vi "Image Version.vi"(6 "Flags":u32=65535 format="%.0x", 8 "error in":errorcluster) -> (0 "error out":errorcluster, 3 "Return":i32)   [LabVIEW 2014]
uses:
  DLL/SDL2.dll
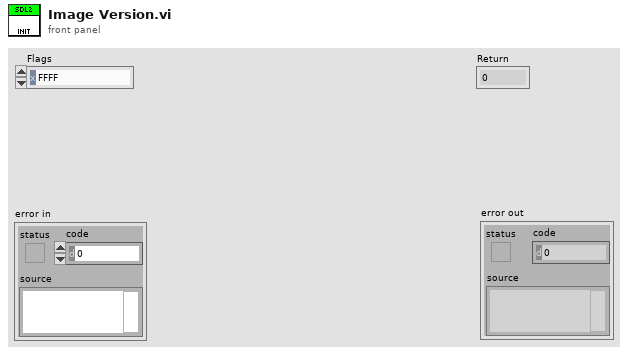
[diagram p1: front panel]
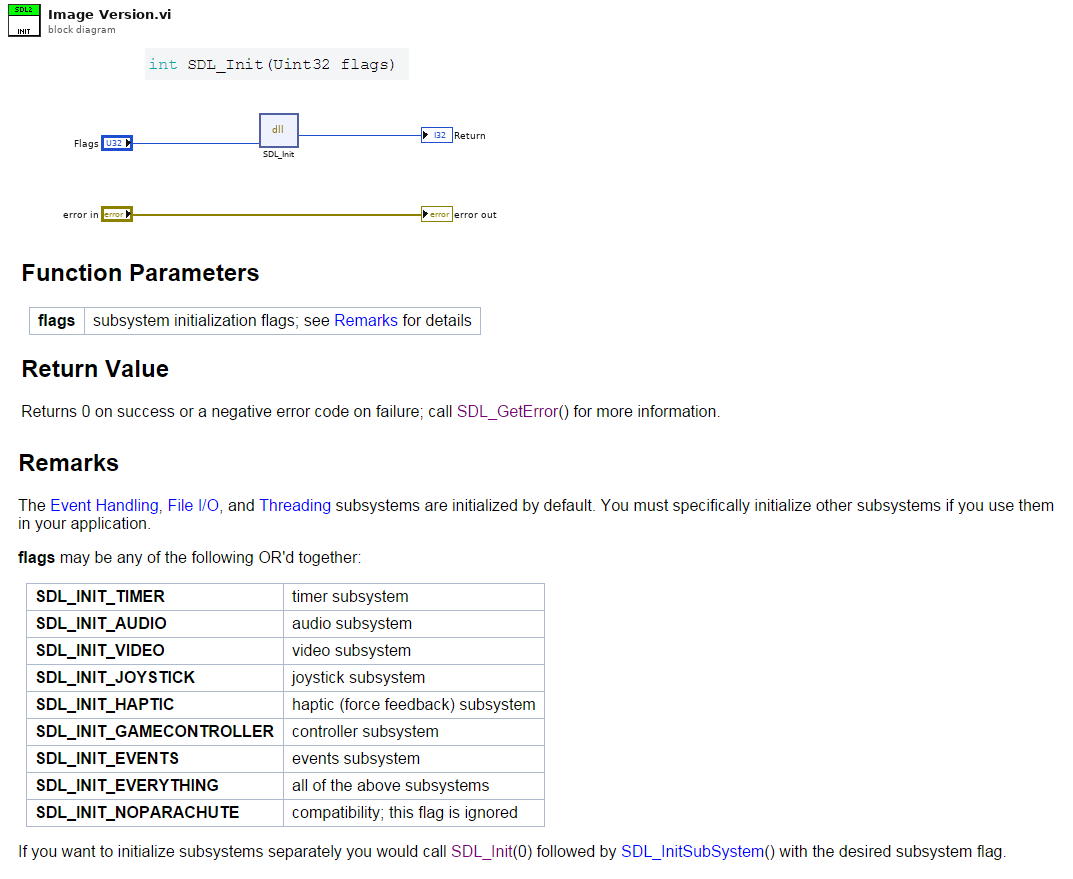
[diagram p0: block diagram]
diagram:
  n1 = dll-call lib="C:/dev/PGS/LabSDL2/Source/LibSDL2 Wrapper/DLL/SDL2.dll" fn="SDL_Init"("flags"="Flags") -> ("return type"=→"Return":i32)  [unwired: 4 in, 2 out]
  "error out" <- "error in"
